vi "Translate gRPC Method FullName.vi"(8 "error in (no error)":errorcluster, 11 "Method Full Name in":string) -> (0 "error out":errorcluster, 3 "Method Full Name out":string)   [LabVIEW 2019, in "gRPC Scripting Tools.lvlib"]
uses:
  gRPC Scripting Tools.lvlib
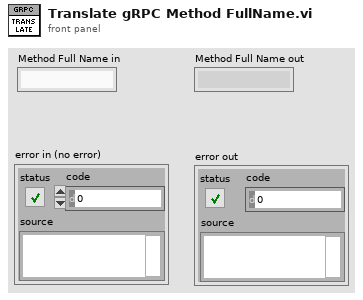
[diagram p1: front panel]
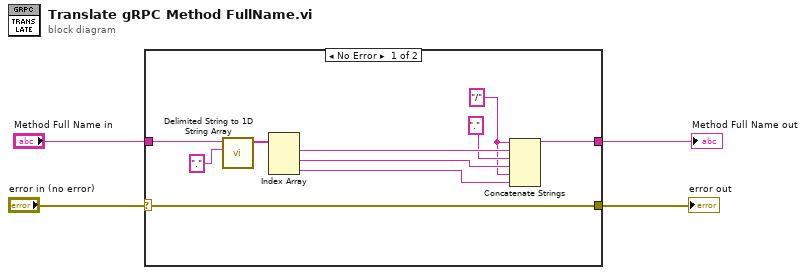
[diagram p0: block diagram]
diagram:
  n1 = case shown="No Error" "error in (no error)" {
    selector: "error in (no error)" -> [w5 w16]
    tunnel: [w14 w15] -> w4
    tunnel: "Method Full Name in" -> [w12 w15]
    tunnel: [w5 w16] -> w1
    frame No Error {
      w7 = "/" ("string")
      n2 = call <vilib>:"Delimited String to 1D String Array.vi"("delimiter"=".", "delimited string"=w12) -> ("string array"=w13:string[])  [unwired: 9 in]
      n3 = Index Array(array=w13) -> (element #1=w10:string, element #2=w8:string, element #3=w6:string)  [unwired: 3 in]
      n4 = Concatenate Strings(w7, w10, "." ("delimiter"), w8, w7, w6) -> (w14:string)
    }
    frame Error {
    }
  }
  "Method Full Name out" <- w4
  "error out" <- w1
